vi "PointMap.vi"(7 "Operation":T2, 8 "error in (no error)":errorcluster, 10 "Map":T1, 11 "Name":string) -> (0 "error out":errorcluster, 1 "All Maps":T1[](array[typedef]), 2 "Map Out":T1, 3 "All Map Names":string[](array[string]), 4 "Found?":bool)   [LabVIEW 2017, in "PointValueMap.lvlib"]
uses:
  <vilib>/addons/PointValueMap/PointValueMap.lvlib
  <vilib>/addons/PointValueMap/controls/PointMapOperations.ctl
  <vilib>/addons/PointValueMap/controls/PointMap.ctl
  <vilib>/addons/PointValueMap/controls/PointMap_Internal.ctl
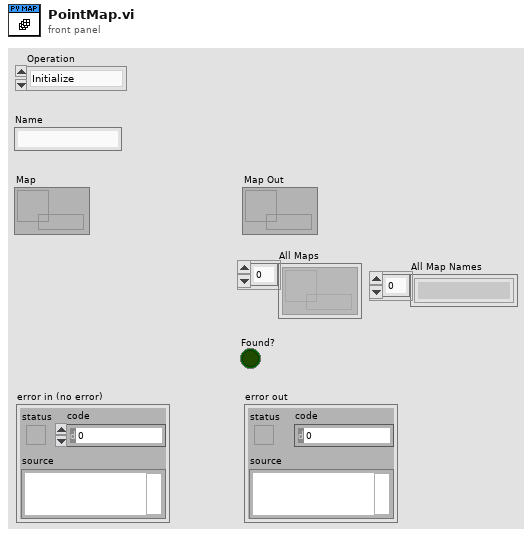
[diagram p1: front panel]
types:
  T1 = typedef "PointValueMap.lvlib/PointMap.ctl" = refnum<data-value>
  T2 = typedef "PointValueMap.lvlib/PointMapOperations.ctl" = enum16{"Initialize", "Create Map", "Update Map", "Get Map", "Get All Maps", "Destroy Map", "Destroy All Maps"}
  T3 = typedef "PointValueMap.lvlib/PointMap_Internal.ctl" = cluster{"Name":string, "Map":T1}
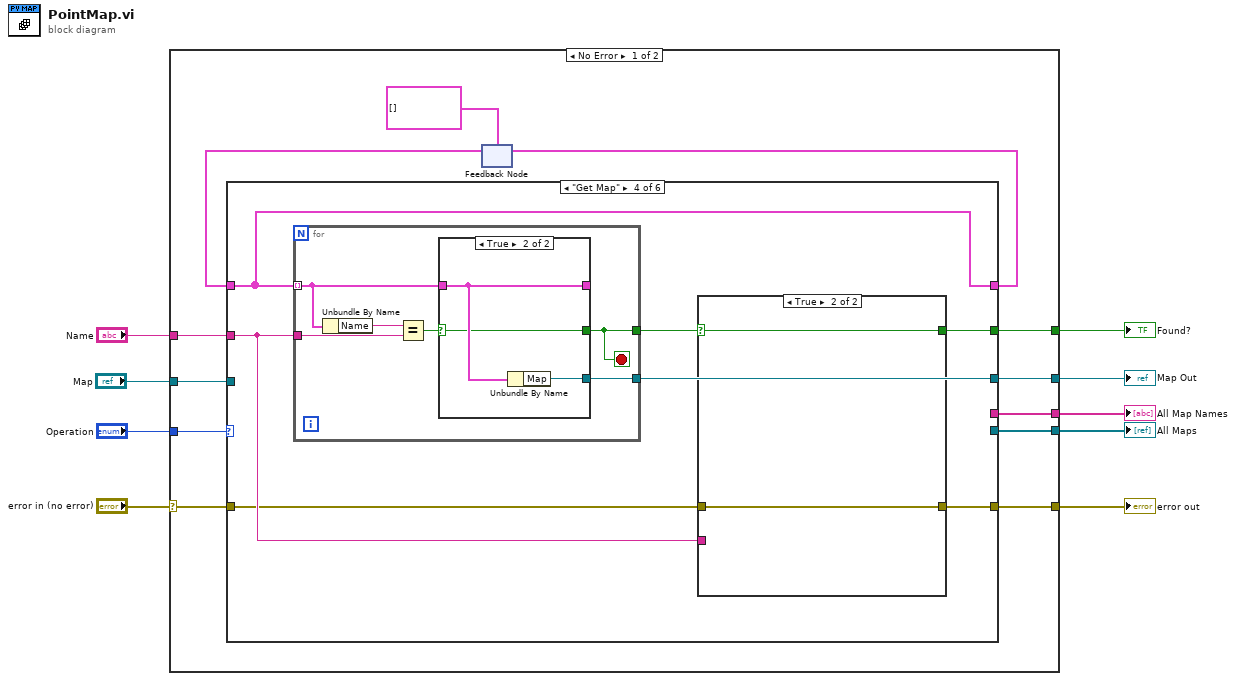
[diagram p0: block diagram]
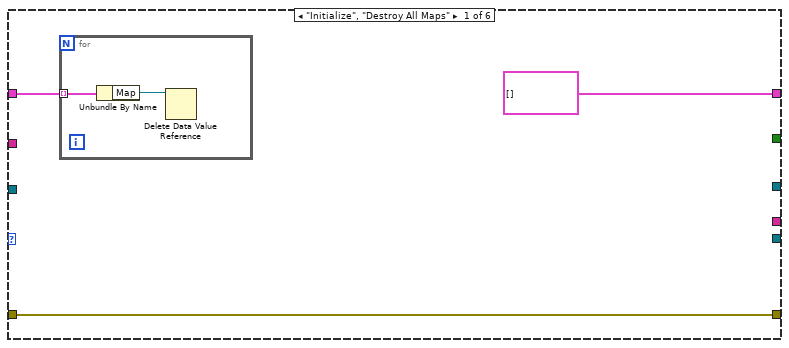
[diagram p2: hidden frame]
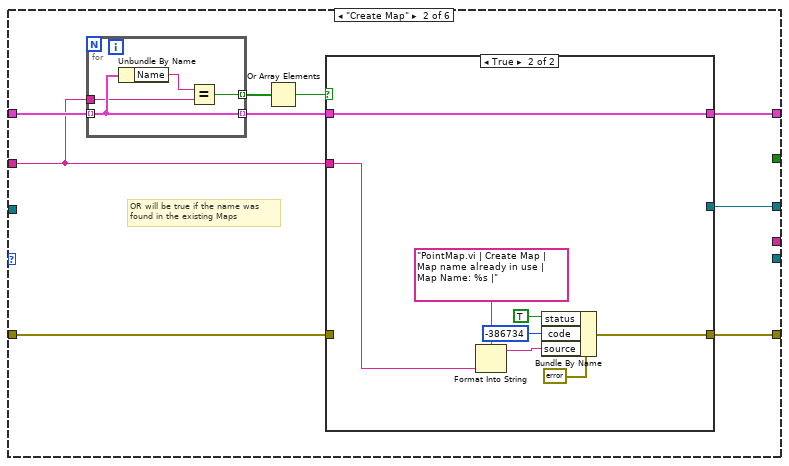
[diagram p3: hidden frame]
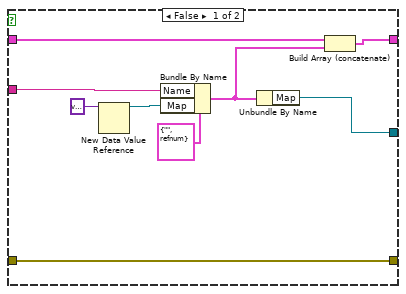
[diagram p4: hidden frame]
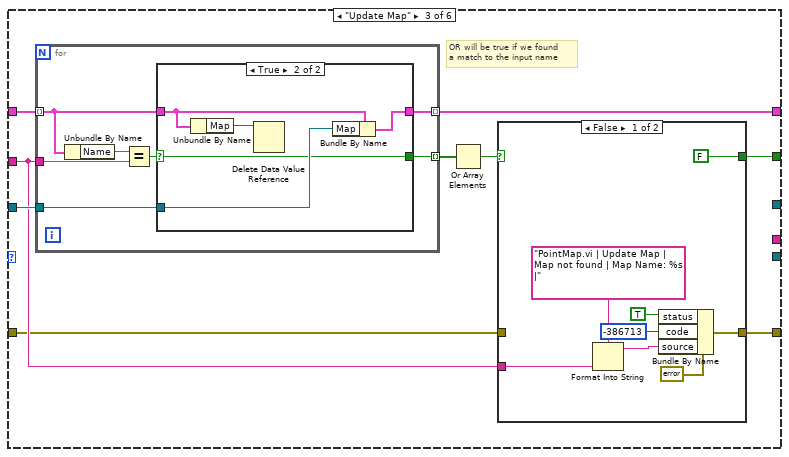
[diagram p5: hidden frame]
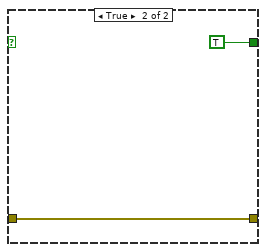
[diagram p6: hidden frame]
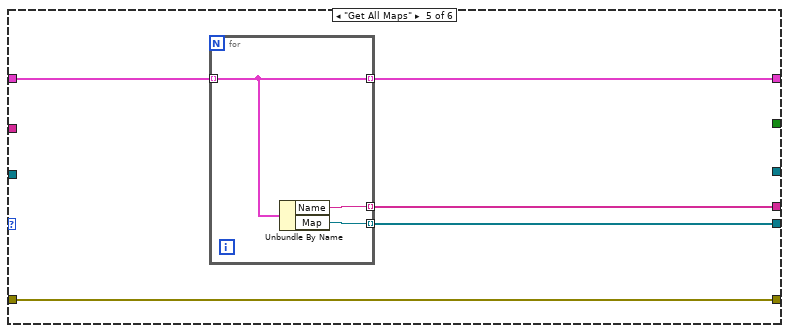
[diagram p10: hidden frame]
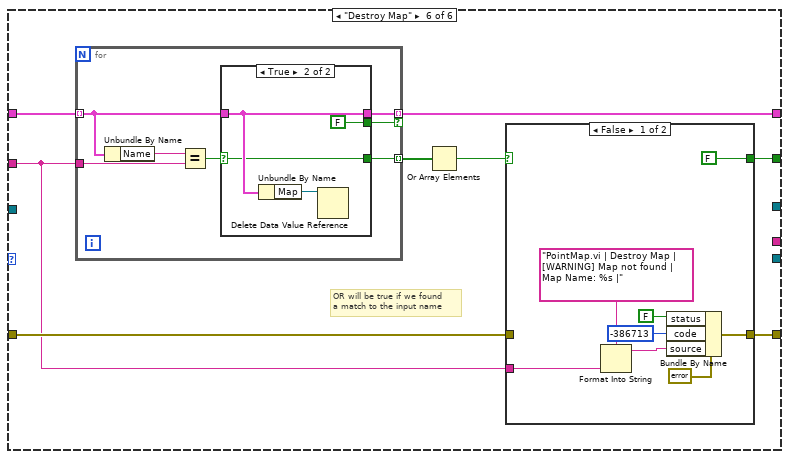
[diagram p11: hidden frame]
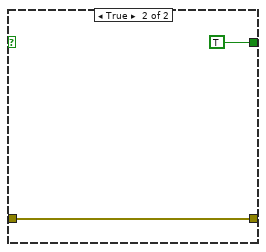
[diagram p12: hidden frame]
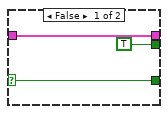
[diagram p13: hidden frame]
diagram:
  n1 = case shown="No Error" "error in (no error)" {
    selector: "error in (no error)" -> [w11 w151]
    tunnel: "Name" -> [w18 _]
    tunnel: [w17 w151] -> w8
    tunnel: [w16 _] -> w7
    tunnel: [w15 _] -> w3
    tunnel: "Operation" -> [w14 _]
    tunnel: "Map" -> [w13 _]
    tunnel: [w12 _] -> w2
    tunnel: [w10 _] -> w1
    frame No Error {
      n2 = feedback #1(T3[] []) -> (w20:T3[])
      n3 = case shown="\"Get Map\"" w14 {
        tunnel: w20 -> [w22 w34 w65 w95 w114 w126]
        tunnel: [T3[] [] w35 w64 w95 w113 w125] -> w19
        tunnel: w18 -> [_ w32 w61 w92 _ w121]
        tunnel: [w23 w29 w57 w90 w115 w123] -> w17
        tunnel: w11 -> [w23 w28 w58 w91 w115 w122]
        tunnel: [_ w27 _ w96 _ _] -> w15
        tunnel: [_ _ w62 w93 _ w124] -> w16
        tunnel: w13 -> [_ _ w63 _ _ _]
        tunnel: [_ _ _ _ w112 _] -> w12
        tunnel: [_ _ _ _ w111 _] -> w10
        frame "Initialize", "Destroy All Maps" {
          n4 = for {
            tunnel: w22 -> [w26] mode=indexing
            n5 = Unbundle By Name(w26) -> ("Map"=w25:T1)
            n6 = Delete Data Value Reference(data value reference=w25) -> ()  [unwired: 1 in, 2 out]
          }
        }
        frame "Create Map" {
          # "OR will be true if the name was\nfound in the existing Maps"
          n7 = for {
            tunnel: [w56] -> w33 mode=indexing
            tunnel: w34 -> [w56] mode=indexing
            tunnel: w32 -> [w54]
            tunnel: [w53] -> w31 mode=indexing
            n8 = Unbundle By Name(w56) -> ("Name"=w55:string)
            n9 = Equal?(x=w55, y=w54) -> (x = y?=w53:bool)
          }
          n10 = Or Array Elements(Boolean array=w31) -> (logical OR=w30:bool)
          n11 = case shown="True" w30 {
            tunnel: [w42 w52] -> w35
            tunnel: w33 -> [w41 w52]
            tunnel: w32 -> [w40 w45]
            tunnel: [w39 w46] -> w29
            tunnel: w28 -> [w39 _]
            tunnel: [w36 _] -> w27
            frame False {
              n12 = New Data Value Reference(data value=variant) -> (data value reference=w37:refnum<data-value>)  [unwired: 1 in, 1 out]
              n13 = Bundle By Name(cluster=T3 {"Name"="", "Map"=refnum} ("Point Map"), "Name"=w40, "Map"=w37) -> (w38:T3)
              n14 = Unbundle By Name(w38) -> ("Map"=w36:T1)
              n15 = Build Array (concatenate)(w41, w38) -> (w42:T3[])
            }
            frame True {
              n16 = Format Into String(format string="PointMap.vi | Create Map | Map name already in use | Map Name: %s |" ("source"), w45) -> (resulting string=w50:string)  [unwired: 2 in, 1 out]
              n17 = Bundle By Name(cluster=errorcluster {"status"=FALSE, "code"=0, "source"=""} ("Error Out"), "status"=TRUE, "code"=-386734, "source"=w50) -> (w46:errorcluster)
            }
          }
        }
        frame "Update Map" {
          # "OR will be true if we found\na match to the input name"
          n18 = for {
            tunnel: w65 -> [w79] mode=indexing
            tunnel: w61 -> [w81]
            tunnel: [w78] -> w64 mode=indexing
            tunnel: w63 -> [w77]
            tunnel: [w76] -> w59 mode=indexing
            n19 = Unbundle By Name(w79) -> ("Name"=w82:string)
            n20 = Equal?(x=w82, y=w81) -> (x = y?=w80:bool)
            n21 = case shown="True" w80 {
              selector: w80 -> [w83 w85]
              tunnel: w79 -> [w84 w87]
              tunnel: [w84 w89] -> w78
              tunnel: w77 -> [_ w88]
              tunnel: [w83 w85] -> w76
              frame False {
              }
              frame True {
                n22 = Unbundle By Name(w87) -> ("Map"=w86:T1)
                n23 = Delete Data Value Reference(data value reference=w86) -> ()  [unwired: 1 in, 2 out]
                n24 = Bundle By Name(cluster=w87, "Map"=w88) -> (w89:T3)
              }
            }
          }
          n25 = Or Array Elements(Boolean array=w59) -> (logical OR=w60:bool)
          n26 = case shown="False" w60 {
            tunnel: [FALSE TRUE] -> w62
            tunnel: [w67 w74] -> w57
            tunnel: w61 -> [w66 _]
            tunnel: w58 -> [_ w74]
            frame False {
              n27 = Format Into String(format string="PointMap.vi | Update Map | Map not found | Map Name: %s |" ("source"), w66) -> (resulting string=w71:string)  [unwired: 2 in, 1 out]
              n28 = Bundle By Name(cluster=errorcluster {"status"=FALSE, "code"=0, "source"=""} ("Error Out"), "status"=TRUE, "code"=-386713, "source"=w71) -> (w67:errorcluster)
            }
            frame True {
            }
          }
        }
        frame "Get Map" {
          n29 = for {
            tunnel: w95 -> [w103] mode=indexing
            tunnel: w92 -> [w105]
            tunnel: [w102] -> w96
            tunnel: [w101] -> w94
            stop <- w101 stop-if-true
            n30 = Unbundle By Name(w103) -> ("Name"=w106:string)
            n31 = Equal?(x=w106, y=w105) -> (x = y?=w104:bool)
            n32 = case shown="True" w104 {
              selector: w104 -> [_ w108]
              tunnel: w103 -> [w107 w110]
              tunnel: [w107 w110] -> _
              tunnel: [_ w109] -> w102
              tunnel: [_ w108] -> w101
              frame False {
              }
              frame True {
                n33 = Unbundle By Name(w110) -> ("Map"=w109:T1)
              }
            }
          }
          n34 = case shown="True" w94 {
            selector: w94 -> [w98 w100]
            tunnel: [w97 w99] -> w90
            tunnel: w92 -> [_ _]
            tunnel: [w98 w100] -> w93
            tunnel: w91 -> [w97 w99]
            frame False {
            }
            frame True {
            }
          }
        }
        frame "Get All Maps" {
          n35 = for {
            tunnel: w114 -> [w118] mode=indexing
            tunnel: [w118] -> w113 mode=indexing
            tunnel: [w117] -> w112 mode=indexing
            tunnel: [w116] -> w111 mode=indexing
            n36 = Unbundle By Name(w118) -> ("Name"=w116:string, "Map"=w117:T1)
          }
        }
        frame "Destroy Map" {
          # "OR will be true if we found\na match to the input name"
          n37 = for {
            tunnel: w126 -> [w140] mode=indexing
            tunnel: w121 -> [w142]
            tunnel: [w139] -> w125 mode=indexing if=w138
            tunnel: [w137] -> w120 mode=indexing
            n38 = Unbundle By Name(w140) -> ("Name"=w143:string)
            n39 = Equal?(x=w143, y=w142) -> (x = y?=w141:bool)
            n40 = case shown="True" w141 {
              selector: w141 -> [w144 w147]
              tunnel: w140 -> [w146 w148]
              tunnel: [w146 w148] -> w139
              tunnel: [TRUE FALSE] -> w138
              tunnel: [w144 w147] -> w137
              frame False {
              }
              frame True {
                n41 = Unbundle By Name(w148) -> ("Map"=w149:T1)
                n42 = Delete Data Value Reference(data value reference=w149) -> ()  [unwired: 1 in, 2 out]
              }
            }
          }
          n43 = Or Array Elements(Boolean array=w120) -> (logical OR=w119:bool)
          n44 = case shown="False" w119 {
            tunnel: [FALSE TRUE] -> w124
            tunnel: [w128 w136] -> w123
            tunnel: w122 -> [_ w136]
            tunnel: w121 -> [w127 _]
            frame False {
              n45 = Format Into String(format string="PointMap.vi | Destroy Map | [WARNING] Map not found | Map Name: %s |" ("source"), w127) -> (resulting string=w132:string)  [unwired: 2 in, 1 out]
              n46 = Bundle By Name(cluster=errorcluster {"status"=FALSE, "code"=0, "source"=""} ("Error Out"), "status"=FALSE, "code"=-386713, "source"=w132) -> (w128:errorcluster)
            }
            frame True {
            }
          }
        }
      }
      n47 = feedback-in #1(w19) -> ()
    }
    frame Error {
    }
  }
  "error out" <- w8
  "Found?" <- w7
  "Map Out" <- w3
  "All Maps" <- w2
  "All Map Names" <- w1
